vi "myRIO v1.0 DO Block Write Resource Manager.vi"(7 "Action":enum16{"Get", "Set"}(ring), 10 "DO Resource In":T1 caption="DO (N Samples) Configuration") -> (1 "Action Succeeds":bool, 2 "DO Resource Out":T1 caption="DO (N Samples) Configuration")   [LabVIEW 2021]
uses:
  <vilib>/myRIO/Common/Instrument Driver Framework/myRIO v1.0/DO Block/typedefs/DO Block Configuration.ctl
  <vilib>/myRIO/Common/Instrument Driver Framework/myRIO v1.0/Resource Manager/vis/myRIO v1.0 Block Write Configuration.vi
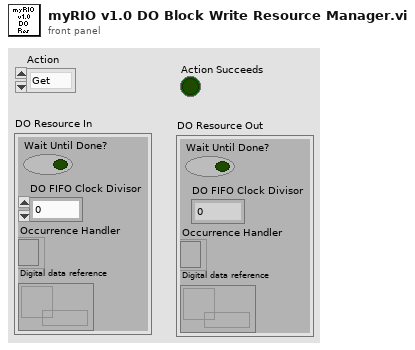
[diagram p1: front panel]
types:
  T1 = typedef "DO Block Configuration.ctl" = cluster{"Wait Until Done?":bool, "DO FIFO Clock Divisor":u16, "Occurrence Handler":refnum<k4>, "Digital data reference":refnum<data-value>}
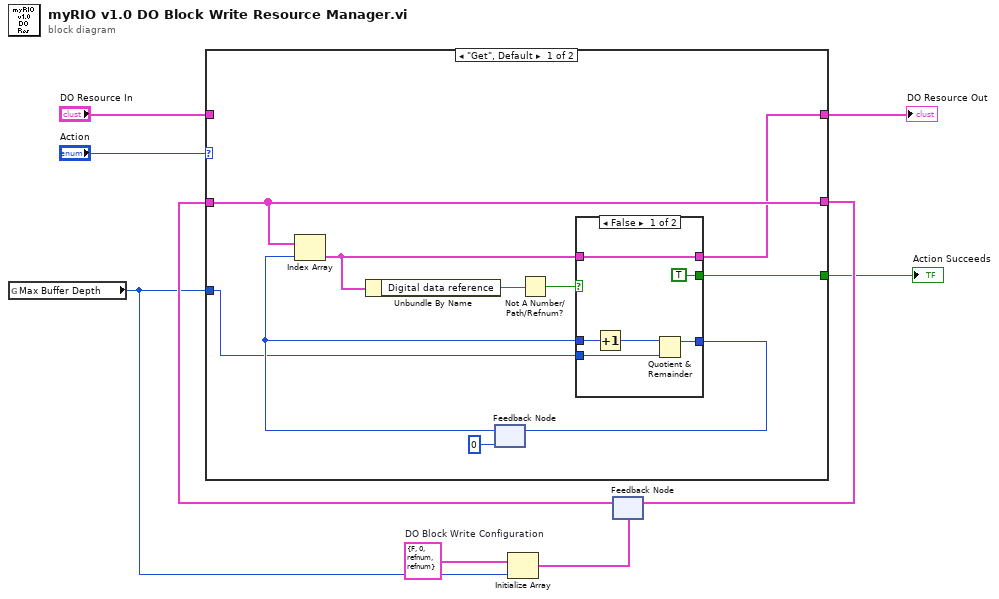
[diagram p0: block diagram]
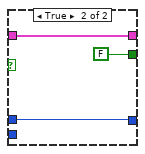
[diagram p2: hidden frame]
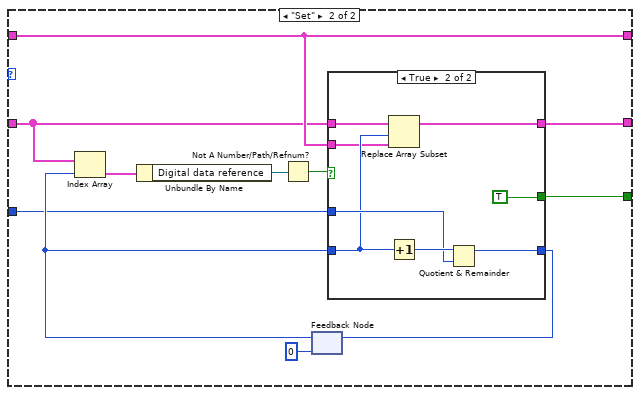
[diagram p3: hidden frame]
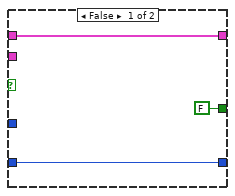
[diagram p4: hidden frame]
diagram:
  w6 = T1 {"Wait Until Done?"=FALSE, "DO FIFO Clock Divisor"=0, "Occurrence Handler"=refnum, "Digital data reference"=refnum}  # DO Block Write Configuration
  n1 = global read "myRIO v1.0 Block Write Configuration.vi" "Max Buffer Depth"() -> (w1:u32)
  n2 = Initialize Array(w6, w1) -> (w5:T1[])
  n3 = feedback #1(w5) -> (w8:T1[])
  n4 = case shown="\"Get\", Default" "Action" {
    tunnel: w8 -> [w13 w32]
    tunnel: "DO Resource In" -> [_ w33]
    tunnel: [w12 w33] -> w4
    tunnel: [w13 w31] -> w3
    tunnel: [w11 w30] -> w2
    tunnel: w1 -> [w10 w29]
    frame "Get", Default {
      n5 = feedback #2(u32 0) -> (w15:u32)
      n6 = Index Array(array=w13, index=w15) -> (element=w16:T1)
      n7 = Unbundle By Name(w16) -> ("Digital data reference"=w18:refnum<data-value>)
      n8 = Not A Number/Path/Refnum?(number/path/refnum=w18) -> (NaN/Path/Refnum?=w17:bool)
      n9 = case shown="False" w17 {
        tunnel: w16 -> [w24 w28]
        tunnel: [w24 w28] -> w12
        tunnel: [TRUE ("Action Succeeds") FALSE ("Action Succeeds")] -> w11
        tunnel: w15 -> [w22 w26]
        tunnel: w10 -> [w21 _]
        tunnel: [w20 w26] -> w14
        frame False {
          n10 = Increment(x=w22) -> (x+1=w23:u32)
          n11 = Quotient & Remainder(x=w23, y=w21) -> (x-y*floor(x/y)=w20:u32)  [unwired: 1 out]
        }
        frame True {
        }
      }
      n12 = feedback-in #2(w14) -> ()
    }
    frame "Set" {
      n13 = feedback #3(u32 0) -> (w35:u32)
      n14 = Index Array(array=w32, index=w35) -> (element=w34:T1)
      n15 = Unbundle By Name(w34) -> ("Digital data reference"=w39:refnum<data-value>)
      n16 = Not A Number/Path/Refnum?(number/path/refnum=w39) -> (NaN/Path/Refnum?=w38:bool)
      n17 = case shown="True" w38 {
        tunnel: w32 -> [w42 w50]
        tunnel: [w42 w49] -> w31
        tunnel: w29 -> [_ w47]
        tunnel: w35 -> [w41 w46]
        tunnel: [w41 w45] -> w36
        tunnel: w33 -> [_ w44]
        tunnel: [FALSE ("Action Succeeds") TRUE ("Action Succeeds")] -> w30
        frame False {
        }
        frame True {
          n18 = Replace Array Subset(array=w50, new element=w44, index=w46) -> (w49:T1[])
          n19 = Increment(x=w46) -> (x+1=w48:u32)
          n20 = Quotient & Remainder(x=w48, y=w47) -> (x-y*floor(x/y)=w45:u32)  [unwired: 1 out]
        }
      }
      n21 = feedback-in #3(w36) -> ()
    }
  }
  "DO Resource Out" <- w4
  "Action Succeeds" <- w2
  n22 = feedback-in #1(w3) -> ()
